vi "Client Spawner.vi"() -> ()   [LabVIEW 2019]
panel:
  in  "# to spawn":i32
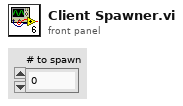
[diagram p1: front panel]
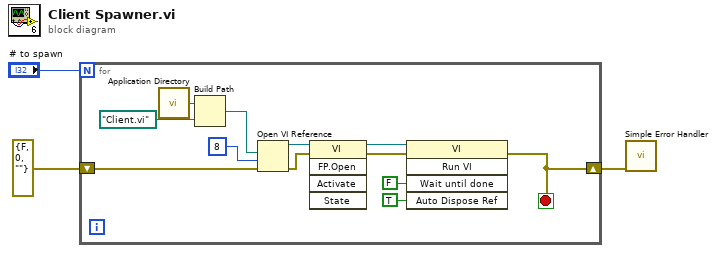
[diagram p0: block diagram]
diagram:
  n1 = for {
    N: "# to spawn" -> [_]
    shift-right: [w4] -> w1
    shift-left: errorcluster {"status"=FALSE, "code"=0, "source"=""} ("error constant") -> [w13]
    stop <- w4 stop-if-true
    n2 = call <vilib>:"Application Directory.vi"() -> ("Application Directory"=w15:path)
    n3 = Build Path(base path=w15, name or relative path=path "Client.vi" ("Application Directory")) -> (appended path=w12:path)
    n4 = Open VI Reference(vi path=w12, options=8, error in (no error)=w13) -> (vi reference=w10:refnum<vi>, error out=w9:errorcluster)  [unwired: 3 in]
    n5 = invoke class="VI" method="FP.Open"(reference=w10, error in=w9) -> (reference out=w8:refnum<vi>, error out=w7:errorcluster)  [unwired: 3 in, 3 out]
    n6 = invoke class="VI" method="Run VI"(reference=w8, error in=w7, "Wait until done"=FALSE ("Wait Until Done"), "Auto Dispose Ref"=TRUE ("Auto Dispose Reference")) -> (error out=w4:errorcluster)  [unwired: 1 in, 4 out]
  }
  n7 = call <vilib>:"Simple Error Handler.vi"("error in (no error)"=w1) -> ()  [unwired: 4 in, 5 out]
